vi "Set Current Limit.vi"(0 "VISA resource name":refnum<visa-resource-name>, 1 "CH number":i32, 2 "Current Limit (5.0 A)":dbl=5.0 caption="Current Limit (5 A)" format="%.2f", 5 "error in (no error)":errorcluster) -> (14 "VISA resource name out":refnum<visa-resource-name>, 19 "error out":errorcluster)   [LabVIEW 2023, in "Rigol.lvlib"]
uses:
  Rigol.lvlib
  <instrlib>/RIGOL DP800 Series/Public/Channels.ctl
  <instrlib>/RIGOL DP800 Series/RIGOL DP800 Series.lvlib
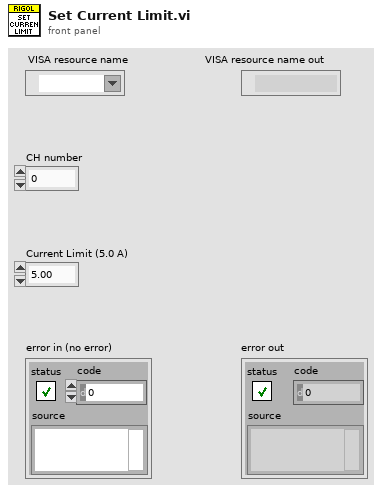
[diagram p1: front panel]
types:
  T1 = typedef "RIGOL DP800 Series.lvlib/Channels.ctl" = i32
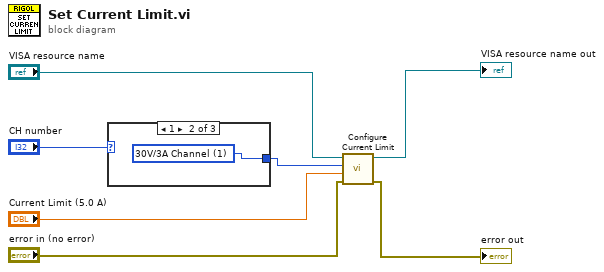
[diagram p0: block diagram]
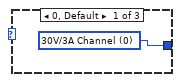
[diagram p2: hidden frame]
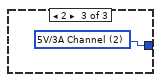
[diagram p3: hidden frame]
diagram:
  n1 = case shown="1" "CH number" {
    tunnel: [w8 w9 w10] -> w2
    frame 0, Default {
      w8 = T1 0 items=["30V/3A Channel", "30V/3A Channel", "5V/3A Channel"] ("Channel (0: 30V Channel)")
    }
    frame 1 {
      w9 = T1 1 items=["30V/3A Channel", "30V/3A Channel", "5V/3A Channel"] ("Channel (0: 30V Channel)")
    }
    frame 2 {
      w10 = T1 2 items=["30V/3A Channel", "30V/3A Channel", "5V/3A Channel"] ("Channel (0: 30V Channel)")
    }
  }
  n2 = call <instrlib>:"Configure Current Limit.vi"("error in (no error)"="error in (no error)", "Current Limit (5.0 A)"="Current Limit (5.0 A)", "Channel (0: 30V Channel)"=w2, "VISA resource name"="VISA resource name") -> ("error out"=→"error out":errorcluster, "VISA resource name out"=→"VISA resource name out":refnum<visa-resource-name>)  [unwired: 6 in]
